vi "packDigital.vi"(8 "error in (no error)":errorcluster, 10 "DigitalOutput":refnum<class "DigitalOutput.lvclass">, 11 "FileReader in":refnum<class "FileReader.lvclass">) -> (0 "error out":errorcluster, 3 "FileReader out":refnum<class "FileReader.lvclass">)   [LabVIEW 2011, in "Tools.lvlib" / "Filing.lvlib" / "FileReader.lvclass"]
uses:
  FileReader.lvclass
  Hal/Channels/Digital/DigitalOutput.lvclass
  FileReader.lvclass/FileReader.ctl
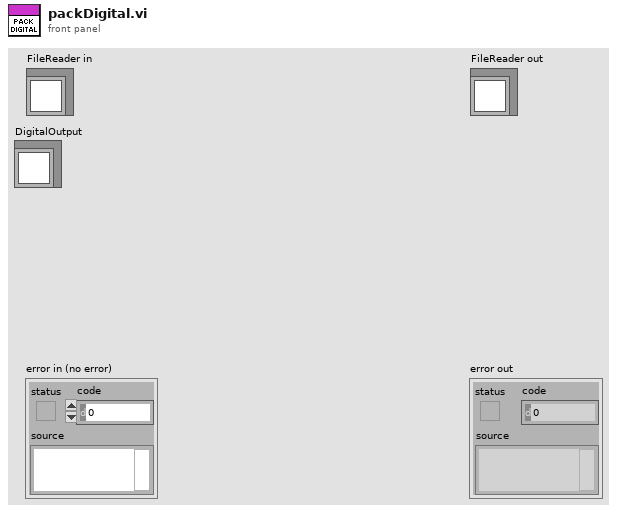
[diagram p1: front panel]
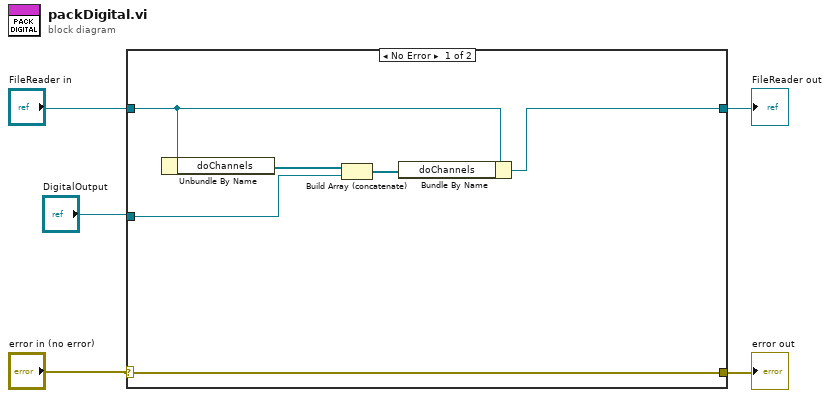
[diagram p0: block diagram]
diagram:
  n1 = case shown="No Error" "error in (no error)" {
    selector: "error in (no error)" -> [w11 w13]
    tunnel: [w11 w13] -> w1
    tunnel: [w6 w12] -> w3
    tunnel: "FileReader in" -> [w8 w12]
    tunnel: "DigitalOutput" -> [w9 _]
    frame No Error {
      n2 = Unbundle By Name(w8) -> ("doChannels"=w10:refnum<class "DigitalOutput.lvclass">[])
      n3 = Build Array (concatenate)(w10, w9) -> (w7:refnum<class "DigitalOutput.lvclass">[])
      n4 = Bundle By Name(cluster=w8, "doChannels"=w7) -> (w6:refnum<class "FileReader.lvclass">)
    }
    frame Error {
    }
  }
  "error out" <- w1
  "FileReader out" <- w3
